vi "rethinkdb_handshake_client_first.vi"(8 "error in (no error)":errorcluster, 10 "password":string, 11 "user":string) -> (0 "error out":errorcluster, 1 "client_first_message":string, 2 "dup password":string, 3 "initial_message":string)   [LabVIEW 2017]
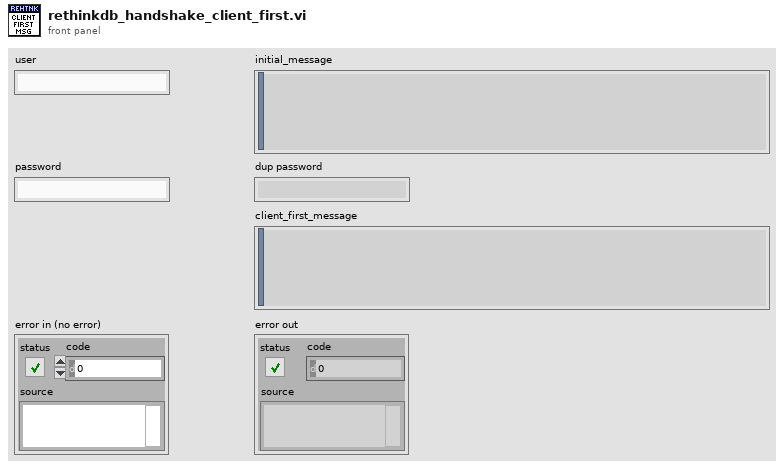
[diagram p1: front panel]
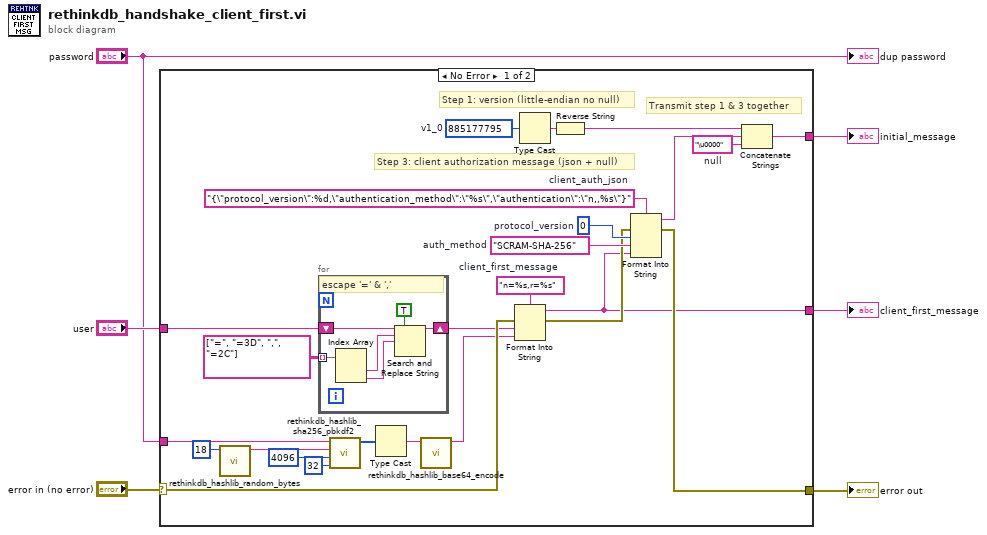
[diagram p0: block diagram]
diagram:
  n1 = case shown="No Error" "error in (no error)" {
    selector: "error in (no error)" -> [w30 w38]
    tunnel: "password" -> [w29 _]
    tunnel: "user" -> [w26 _]
    tunnel: [w10 w38] -> w4
    tunnel: [w17 _] -> w3
    tunnel: [w8 _] -> w2
    frame No Error {
      w12 = "SCRAM-SHA-256"  # auth_method
      w13 = 0  # protocol_version
      w14 = "{\"protocol_version\":%d,\"authentication_method\":\"%s\",\"authentication\":\"n,,%s\"}"  # client_auth_json
      w15 = "\u0000"  # null
      w23 = u32 885177795  # v1_0
      w31 = "n=%s,r=%s"  # client_first_message
      # "Step 3: client authorization message (json + null)"
      # "Transmit step 1 & 3 together"
      # "Step 1: version (little-endian no null)"
      n2 = call "rethinkdb_hashlib_random_bytes.vi"("length (18bytes)"=18 ("length")) -> ("random bytes"=w19:string)  [unwired: 10 in]
      n3 = for {
        shift-right: [w36] -> w25
        shift-left: w26 -> [w37]
        tunnel: string[][] [["=", "=3D"], [",", "=2C"]] -> [w34] mode=indexing
        # "escape '=' & ','"
        n4 = Index Array(array=w34) -> (element #1=w33:string, element #2=w32:string)  [unwired: 2 in]
        n5 = Search and Replace String(replace all?=TRUE ("replace all? (F)"), input string=w37, search string=w33, replace string=w32) -> (result string=w36:string)  [unwired: 4 in, 3 out]
      }
      n6 = call "rethinkdb_hashlib_sha256_pbkdf2.vi"("dkLen (32octets=sha256)"=32, "iterations"=4096, "salt"=w19, "password"=w29) -> ("sha-256"=w7:u32[])  [unwired: 7 in]
      n7 = Type Cast(x=w7) -> (*(type *) &x=w28:string)  [unwired: 1 in]
      n8 = call "rethinkdb_hashlib_base64_encode.vi"("string"=w28) -> ("base64"=w27:string)  [unwired: 10 in]
      n9 = Format Into String(format string=w31, error in=w30, w25, w27) -> (resulting string=w8:string, error out=w11:errorcluster)  [unwired: 1 in]
      n10 = Type Cast(x=w23) -> (*(type *) &x=w22:string)  [unwired: 1 in]
      n11 = Reverse String(1:w22) -> (0:w16:string)
      n12 = Format Into String(format string=w14, error in=w11, w13, w12, w8) -> (resulting string=w9:string, error out=w10:errorcluster)  [unwired: 1 in]
      n13 = Concatenate Strings(w16, w9, w15) -> (w17:string)
    }
    frame Error {
    }
  }
  "error out" <- w4
  "initial_message" <- w3
  "client_first_message" <- w2
  "dup password" <- "password"
